vi "Initialize Save Images VI.vi"(8 "error in (no error)":errorcluster, 11 "Channel in":refnum<class "Channel.lvclass">) -> (0 "error out":errorcluster, 3 "Channel out":refnum<class "Channel.lvclass">)   [LabVIEW 2018, in "Channel.lvclass"]
doc: "Run the VI responsible for saving the images"
uses:
  Channel.lvclass
  Channel.lvclass/Channel.ctl
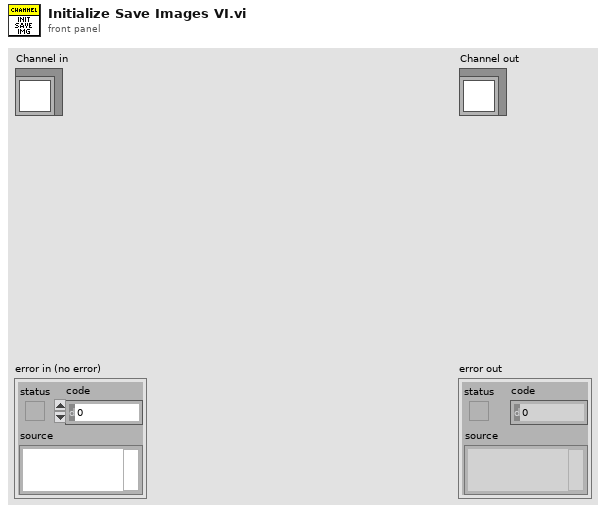
[diagram p1: front panel]
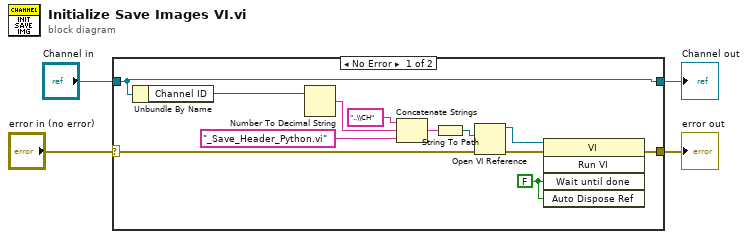
[diagram p0: block diagram]
diagram:
  n1 = case shown="No Error" "error in (no error)" {
    selector: "error in (no error)" -> [w7 w18]
    tunnel: [w12 w18] -> w3
    tunnel: [w6 w17] -> w1
    tunnel: "Channel in" -> [w6 w17]
    frame No Error {
      w15 = FALSE ("Wait Until Done")
      n2 = Unbundle By Name(w6) -> ("Channel ID"=w5:u8)
      n3 = Number To Decimal String(number=w5) -> (decimal integer string=w13:string)  [unwired: 1 in]
      n4 = Concatenate Strings("..\\CH" ("name or relative path"), w13, "_Save_Header_Python.vi" ("name or relative path")) -> (w9:string)
      n5 = String To Path(string=w9) -> (path=w10:path)
      n6 = Open VI Reference(vi path=w10, error in (no error)=w7) -> (vi reference=w16:refnum<vi>, error out=w8:errorcluster)  [unwired: 4 in]
      n7 = invoke class="VI" method="Run VI"(reference=w16, error in=w8, "Wait until done"=w15, "Auto Dispose Ref"=w15) -> (error out=w12:errorcluster)  [unwired: 1 in, 4 out]
    }
    frame Error {
    }
  }
  "error out" <- w3
  "Channel out" <- w1
